vi "kalman measure step not single cycle.vi"(6 "v-feedback?":bool, 7 "vmax":fxp<+,16,0> format="%.32g", 10 "state in":T1={"pos estimate"=-30.139999389648438, "v estimate"=6.103515625e-05, "weighted position error sum"=438.0, "photon count"=64, "transmit tick count"=0, "axis number"=0, "px (levels^2)"=298.0, "pxv (levels^2/ticks)"=0.003100000321865082, "pv (levels^2/ticks^2)"=6.199999802447564e-08, "vel diff (levels^2/ticks^3)"=0.0, "gx"=1.5546875, "rtwiddle"=66560.0, "photon count ch0"=0, "photon count ch1"=0, "Dx -levels^2/ticks"=0.0}) -> (2 "state out":T1)   [LabVIEW 2010]
uses:
  integrating single axis kalman state.ctl
  <vilib>/rvi/FXPMathLib/FxpMul/XNode/nifxpmath_Multiplier.xnode
  <vilib>/rvi/FXPMathLib/FxpMul/subVIs/nifxpmath_Mul_SimConfig.ctl
  <vilib>/fxp/LVFixedPointQuantizationPolicyTypeDef.ctl
  <vilib>/fxp/LVFixedPointOverflowPolicyTypeDef.ctl
  <vilib>/rvi/FXPMathLib/FxpAdd/XNode/nifxpmath_Add.xnode
  <vilib>/rvi/FXPMathLib/FxpAdd/subVIs/nifxpmath_Add_SimConfig.ctl
  <vilib>/rvi/FXPMathLib/FxpReciprocal/XNode/nifxpmath_Reciprocal.xnode
  <vilib>/rvi/FXPMathLib/FxpDiv/XNode/nifxpmath_Div.xnode
  <vilib>/rvi/FXPMathLib/FxpDiv/subVIs/nifxpmath_Div_SimConfig.ctl
  <vilib>/rvi/FXPMathLib/FxpSub/XNode/nifxpmath_Sub.xnode
  <vilib>/rvi/FXPMathLib/FxpSub/subVIs/nifxpmath_Sub_SimConfig.ctl
  <vilib>/rvi/FXPMathLib/FxpMul/simVIs/DllFxpMulTemp_sub.vi
  <vilib>/rvi/FXPMathLib/FxpAdd/simVIs/DllFxpAddTemp_sub.vi
  <vilib>/rvi/FXPMathLib/FxpDiv/simVIs/DllFxpDivTemp_sub.vi
  <vilib>/rvi/FXPMathLib/FxpSub/simVIs/DllFxpSubTemp_sub.vi
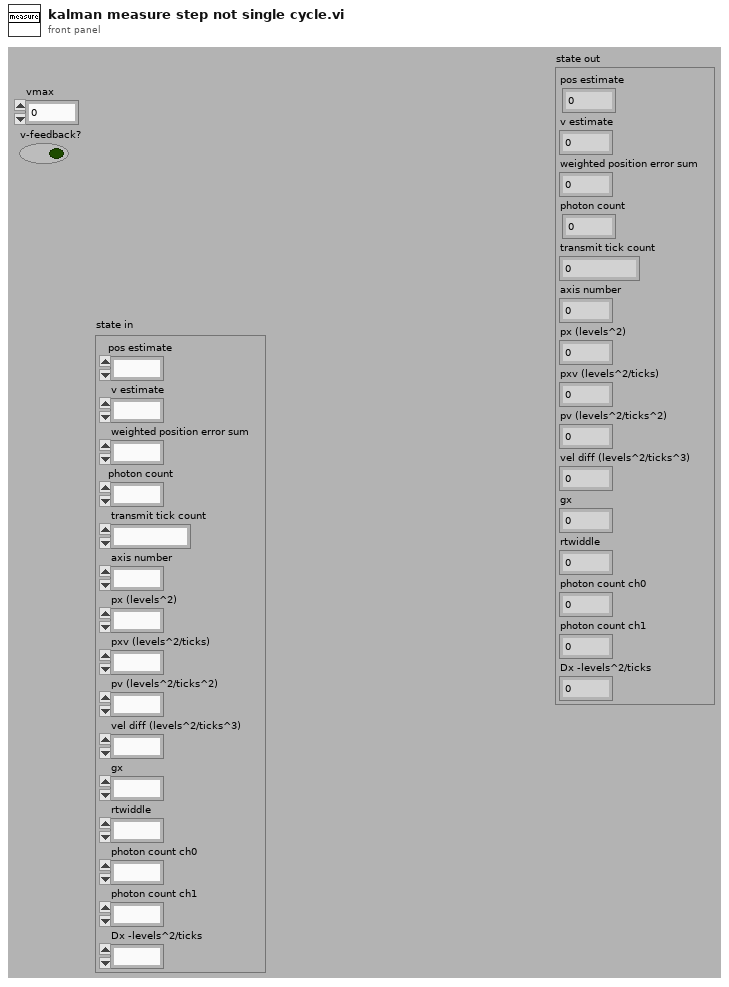
[diagram p1: front panel]
types:
  T1 = typedef "integrating single axis kalman state.ctl" = cluster{"pos estimate":fxp<+/-,32,16>, "v estimate":fxp<+/-,16,0>, "weighted position error sum":fxp<+/-,32,32>, "photon count":u32, "transmit tick count":u32, "axis number":u8, "px (levels^2)":fxp<+,32,19>, "pxv (levels^2/ticks)":fxp<+,32,2>, "pv (levels^2/ticks^2)":fxp<+,32,-14>, "vel diff (levels^2/ticks^3)":fxp<+,24,-22>, "gx":fxp<+,16,8>, "rtwiddle":fxp<+,16,26>, "photon count ch0":u32, "photon count ch1":u32, "Dx -levels^2/ticks":fxp<+,32,19>}
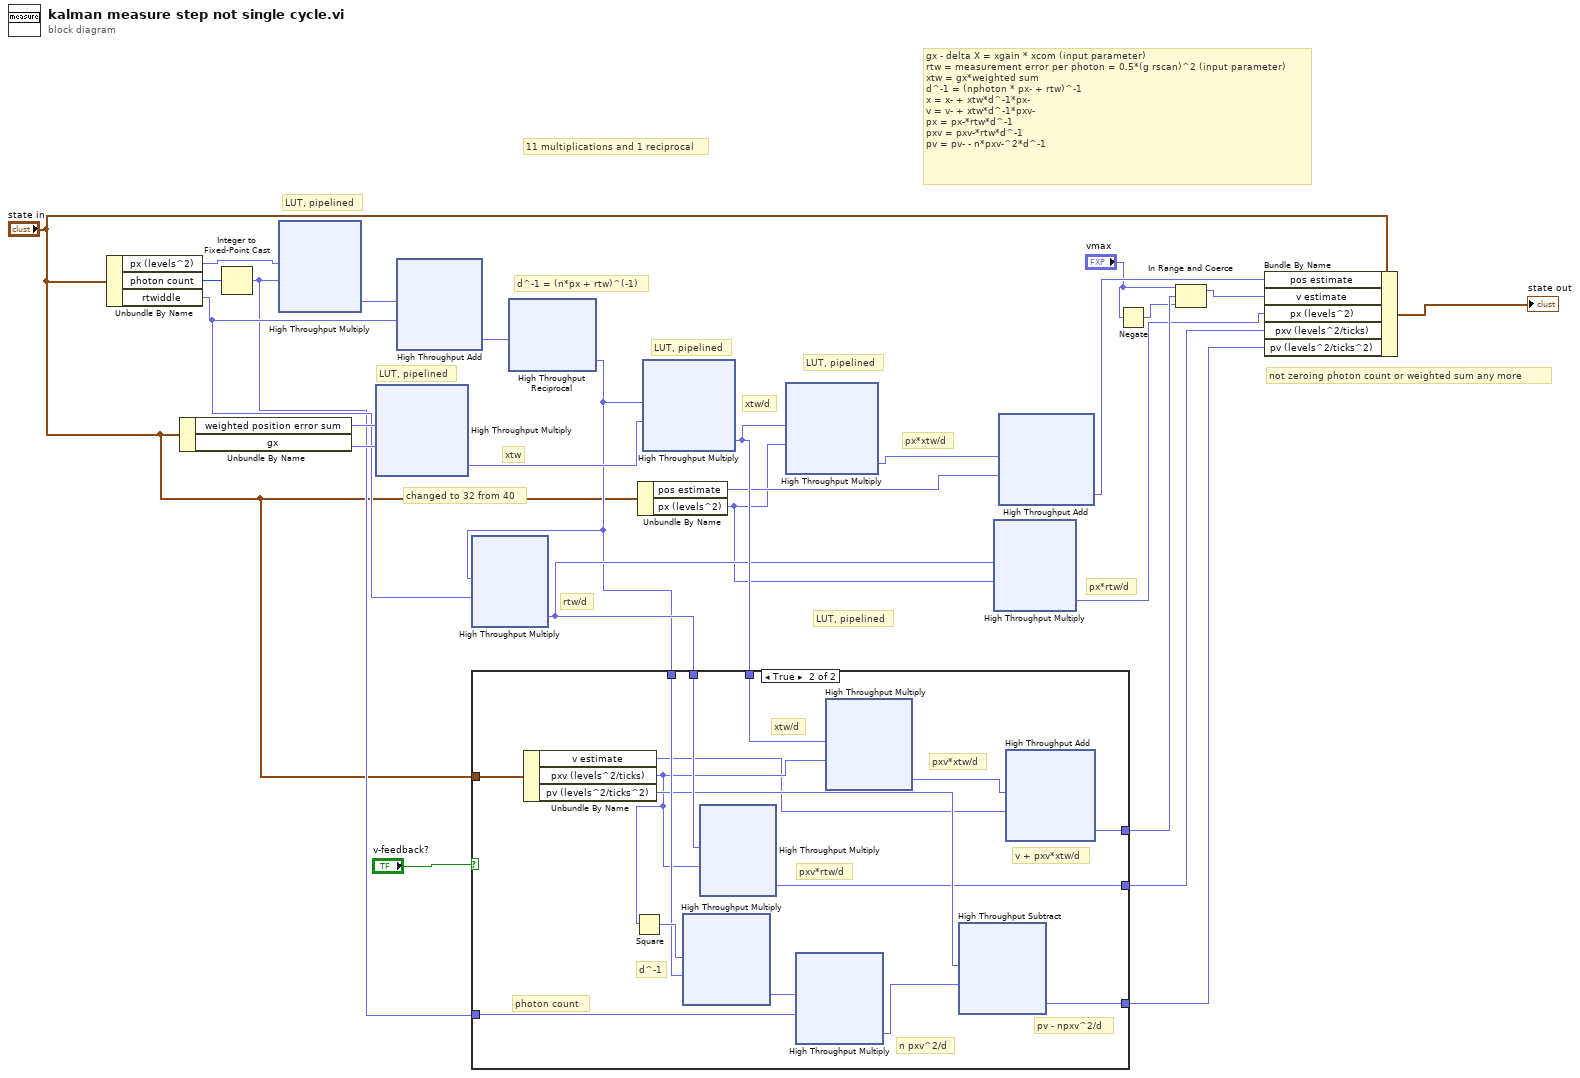
[diagram p0: block diagram]
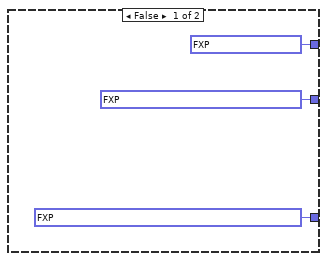
[diagram p2: hidden frame]
diagram:
  # "px*rtw/d"
  # "px*xtw/d"
  # "xtw/d"
  # "xtw"
  # "not zeroing photon count or weighted sum any more"
  # "LUT, pipelined"
  # "LUT, pipelined"
  # "changed to 32 from 40"
  # "LUT, pipelined"
  # "LUT, pipelined"
  # "LUT, pipelined"
  # "gx - delta X = xgain * xcom (input parameter)\nrtw = measurement error per photon = 0.5*(g rscan)^2 (input parameter)\nxtw = gx*weighted sum\nd^-1 = (nphoton * px- + rtw)^-1\nx = x- + xtw*d^-1*px-\nv = v- + xtw*d^-1*pxv-\npx = px-*rtw*d^-1\npxv = pxv-*rtw*d^-1\npv = pv- - n*pxv-^2*d^-1"
  # "11 multiplications and 1 reciprocal"
  # "rtw/d"
  # "d^-1 = (n*px + rtw)^(-1)"
  n1 = Unbundle By Name("state in") -> ("px (levels^2)"=w25:fxp<+,32,19>, "photon count"=w26:u32, "rtwiddle"=w16:fxp<+,16,26>)
  n2 = Unbundle By Name("state in") -> ("weighted position error sum"=w22:fxp<+/-,32,32>, "gx"=w21:fxp<+,16,8>)
  n3 = Integer to Fixed-Point Cast(integer=w26) -> (fixed-point=w13:fxp<+,32,32>)  [unwired: 1 in]
  n4 = xnode "High Throughput Multiply"("x"=w25, "y"=w13) -> ("x*y"=w24:fxp<+,32,42>)
  n5 = xnode "High Throughput Multiply"("x"=w22, "y"=w21) -> ("x*y"=w20:fxp<+/-,32,32>)
  n6 = xnode "High Throughput Add"("x"=w24, "y"=w16) -> ("x+y"=w23:fxp<+,32,42>)
  n7 = xnode "High Throughput Reciprocal"("x"=w23) -> ("1/x"=w14:fxp<+,32,-10>)
  n8 = xnode "High Throughput Multiply"("x"=w14, "y"=w16) -> ("x*y"=w15:fxp<+,32,0>)
  n9 = Unbundle By Name("state in") -> ("pos estimate"=w17:fxp<+/-,32,16>, "px (levels^2)"=w2:fxp<+,32,19>)
  n10 = xnode "High Throughput Multiply"("x"=w14, "y"=w20) -> ("x*y"=w19:fxp<+/-,32,11>)
  n11 = case shown="True" "v-feedback?" {
    tunnel: w19 -> [_ w44]
    tunnel: w15 -> [_ w42]
    tunnel: w14 -> [_ w40]
    tunnel: w13 -> [_ w38]
    tunnel: [fxp<+/-,16,0> 0.0 ("x+y") w35] -> w11
    tunnel: [fxp<+,32,2> 0.0 ("x*y") w34] -> w9
    tunnel: [fxp<+,32,-14> 0.0 ("x-y") w33] -> w8
    tunnel: "state in" -> [_ w32]
    frame False {
    }
    frame True {
      # "pv - npxv^2/d"
      # "pxv*rtw/d"
      # "d^-1"
      # "n pxv^2/d"
      # "v + pxv*xtw/d"
      # "pxv*xtw/d"
      # "xtw/d"
      # "photon count"
      n12 = Unbundle By Name(w32) -> ("v estimate"=w30:fxp<+/-,16,0>, "pxv (levels^2/ticks)"=w31:fxp<+,32,2>, "pv (levels^2/ticks^2)"=w37:fxp<+,32,-14>)
      n13 = Square(x=w31) -> (x^2=w41:fxp<+,32,4>)
      n14 = xnode "High Throughput Multiply"("x"=w41, "y"=w40) -> ("x*y"=w39:fxp<+,32,-14>)
      n15 = xnode "High Throughput Multiply"("x"=w42, "y"=w31) -> ("x*y"=w34:fxp<+,32,2>)
      n16 = xnode "High Throughput Multiply"("x"=w39, "y"=w38) -> ("x*y"=w36:fxp<+,32,-14>)
      n17 = xnode "High Throughput Multiply"("x"=w44, "y"=w31) -> ("x*y"=w43:fxp<+/-,16,0>)
      n18 = xnode "High Throughput Subtract"("x"=w37, "y"=w36) -> ("x-y"=w33:fxp<+,32,-14>)
      n19 = xnode "High Throughput Add"("x"=w43, "y"=w30) -> ("x+y"=w35:fxp<+/-,16,0>)
    }
  }
  n20 = xnode "High Throughput Multiply"("x"=w19, "y"=w2) -> ("x*y"=w18:fxp<+/-,32,16>)
  n21 = xnode "High Throughput Multiply"("x"=w15, "y"=w2) -> ("x*y"=w10:fxp<+,32,19>)
  n22 = xnode "High Throughput Add"("x"=w18, "y"=w17) -> ("x+y"=w12:fxp<+/-,32,16>)
  n23 = Negate(x="vmax") -> (-x=w4:fxp<+/-,16,0>)
  n24 = In Range and Coerce(upper limit="vmax", x=w11, lower limit=w4) -> (coerced(x)=w6:fxp<+/-,17,1>)  [unwired: 1 out]
  n25 = Bundle By Name(cluster="state in", "pos estimate"=w12, "v estimate"=w6, "px (levels^2)"=w10, "pxv (levels^2/ticks)"=w9, "pv (levels^2/ticks^2)"=w8) -> (→"state out":T1)
